vi "Path2.vi"(8 "error in (no error)":errorcluster, 11 "KNR in":T2) -> (0 "error out 4":errorcluster caption="error out", 1 "Number of Matches (Shape Detection 1)":i32, 2 "Circles (Shape Detection 1)":T1(array[cluster]) {"Position"."Y" format="%.2f"; "Position"."X" format="%.2f"}, 3 "KNR out":T2, 5 "Pcmd":dbl)   [LabVIEW 2013]
uses:
  <userlib>/KNR OS 3.0 LabVIEW Toolkit/Type Definition/KNR3 Reference.ctl
  <userlib>/_FPGA Interface Advanced Tools/FPGA Interface Base/FPGA Interface Base.lvclass
  <userlib>/KNR OS 3.0 LabVIEW Toolkit/Type Definition/Resource.ctl
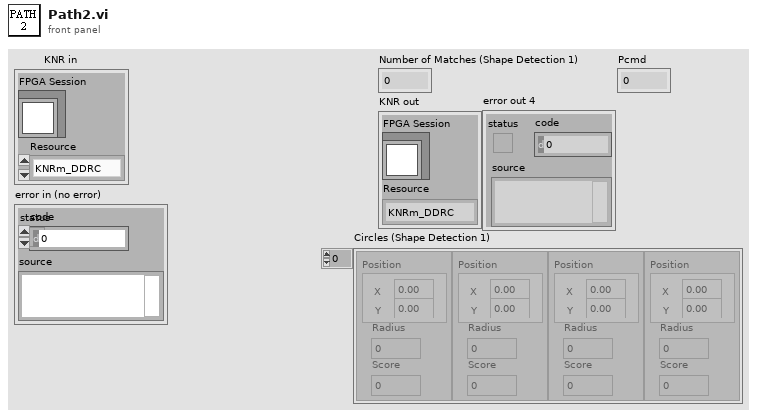
[diagram p1: front panel]
types:
  T1 = cluster{"Position":cluster{"X":sgl, "Y":sgl}, "Radius":dbl, "Score":dbl}[]
  T2 = typedef "KNR3 Reference.ctl" = cluster{"FPGA Session":refnum<class "FPGA Interface Base.lvclass">, "Resource":T3}
  T3 = typedef "Resource.ctl" = enum16{"KNRm_DDRC", "KNRm_DDDD", "KNRm_DDDR", "KNRm_DDDC", "KNR"}
  T4 = cluster{"Mode":enum16{"FRWD", "TURFIX", "TURNOF", "CIRCULAR"}, "Dir":enum16{"Left", "Right"}, "Pcmd":dbl, "Vcmd":dbl, "X":dbl, "Y":dbl}
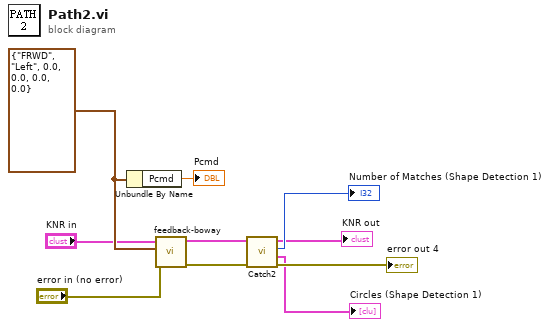
[diagram p0: block diagram]
diagram:
  w10 = T4 {"Mode"=enum."FRWD", "Dir"=enum."Left", "Pcmd"=0.0, "Vcmd"=0.0, "X"=0.0, "Y"=0.0} ("Move")
  n1 = Unbundle By Name(w10) -> ("Pcmd"=→"Pcmd":dbl)
  n2 = call "feedback-boway.vi"("error in (no error)"="error in (no error)", "Move"=w10, "KNR in"="KNR in") -> ("error out"=w5:errorcluster, "KNR out"=w6:T2)  [unwired: 6 in, 1 out]
  n3 = call "Catch2.vi"("Error"=w5, "KNR in"=w6) -> ("error out 4"=→"error out 4":errorcluster, "Circles (Shape Detection 1)"=→"Circles (Shape Detection 1)":T1, "Number of Matches (Shape Detection 1)"=→"Number of Matches (Shape Detection 1)":i32, "KNR out"=→"KNR out":T2)  [unwired: 5 in, 1 out]
